vi "01_MakeArray.vi"(0 "Amp":dbl, 1 "Step":dbl) -> (7 "Array":dbl[](array[numeric]))   [LabVIEW 2017]
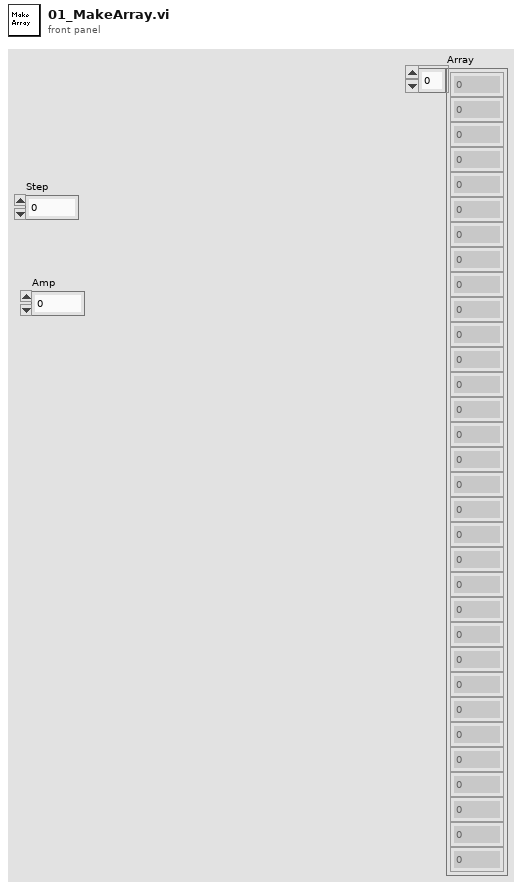
[diagram p1: front panel]
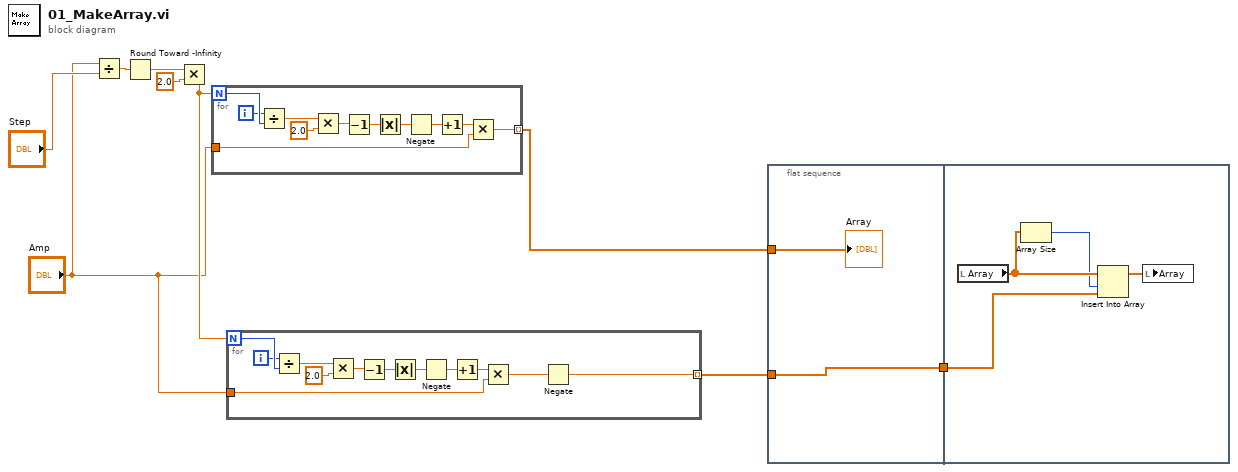
[diagram p0: block diagram]
diagram:
  n1 = Divide(x="Amp", y="Step") -> (x/y=w6:dbl)
  n2 = Round Toward -Infinity(1:w6) -> (0:w7:dbl)
  n3 = Multiply(x=w7, y=2.0) -> (x*y=w5:dbl)
  n4 = for {
    N: w5 -> [w20]
    tunnel: "Amp" -> [w11]
    tunnel: [w10] -> w3 mode=indexing
    i -> [w19]
    n5 = Divide(x=w19, y=w20) -> (x/y=w18:dbl)
    n6 = Multiply(x=w18, y=2.0) -> (x*y=w16:dbl)
    n7 = Decrement(x=w16) -> (x-1=w15:dbl)
    n8 = Absolute Value(x=w15) -> (abs(x)=w14:dbl)
    n9 = Negate(x=w14) -> (-x=w13:dbl)
    n10 = Increment(x=w13) -> (x+1=w12:dbl)
    n11 = Multiply(x=w12, y=w11) -> (x*y=w10:dbl)
  }
  n12 = for {
    N: w5 -> [w32]
    tunnel: "Amp" -> [w23]
    tunnel: [w21] -> w1 mode=indexing
    i -> [w31]
    n13 = Divide(x=w31, y=w32) -> (x/y=w30:dbl)
    n14 = Multiply(x=w30, y=2.0) -> (x*y=w28:dbl)
    n15 = Decrement(x=w28) -> (x-1=w27:dbl)
    n16 = Absolute Value(x=w27) -> (abs(x)=w26:dbl)
    n17 = Negate(x=w26) -> (-x=w25:dbl)
    n18 = Increment(x=w25) -> (x+1=w24:dbl)
    n19 = Multiply(x=w24, y=w23) -> (x*y=w22:dbl)
    n20 = Negate(x=w22) -> (-x=w21:dbl)
  }
  n21 = flat-sequence {
    tunnel: w3 -> [w34]
    tunnel: [w33] -> w2
    tunnel: w1 -> [w33]
    tunnel: w2 -> [w36]
    frame #0 {
      "Array" <- w34
    }
    frame #1 {
      n22 = local read "Array"() -> (w37:dbl[])
      n23 = Array Size(array=w37) -> (size(s)=w35:i32)
      n24 = Insert Into Array(array=w37, index=w35, new element=w36) -> (w38:dbl[])
      n25 = local write "Array"(w38) -> ()
    }
  }
